vi "getAzimuth.vi"(8 "error in (no error)":errorcluster, 11 "IDome in":refnum<class "IDome.lvclass">) -> (0 "error out":errorcluster, 2 "azimuth":T1 min=0.0 max=360.0, 3 "IDome out":refnum<class "IDome.lvclass">)   [LabVIEW 2016, in "IDome.lvclass"]
uses:
  IDome.lvclass
  domeTypedefs/azimuth.ctl
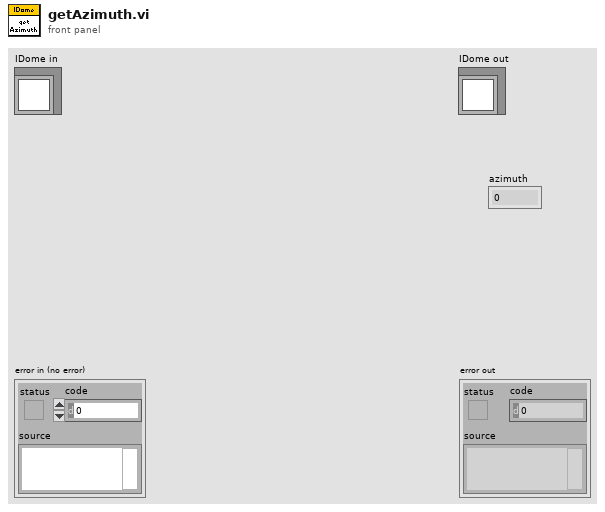
[diagram p1: front panel]
types:
  T1 = typedef "azimuth.ctl" = dbl
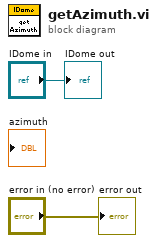
[diagram p0: block diagram]
diagram:
  "error out" <- "error in (no error)"
  "IDome out" <- "IDome in"
